vi "JSON Alarmas.vi"(0 "time":u32, 1 "high bat":dbl, 2 "Fault Modul":dbl, 5 "Temperatura":dbl, 7 "Common Sys":dbl, 9 "out line 1":dbl, 11 "error in":errorcluster, 12 "out line 3":dbl, 13 "low bat":dbl) -> (4 "alarmas":refnum<class "JSON Array.lvclass">, 15 "error out":errorcluster)   [LabVIEW 2015]
uses:
  <vilib>/addons/JSON API/Get Polymorphic/JSON GetSet.lvlib
  <vilib>/addons/JSON API/JSON Scalar/Set SGL.vi
  <vilib>/addons/JSON API/JSON Scalar/JSON Scalar.lvclass
  <vilib>/addons/JSON API/JSON Object/Set Object Item by name.vi
  <vilib>/addons/JSON API/JSON Object/JSON Object.lvclass
  <vilib>/addons/JSON API/JSON Scalar/Set String.vi
  <vilib>/addons/JSON API/JSON Array/Set JSON Array.vi
  <vilib>/addons/JSON API/JSON Array/JSON Array.lvclass
  <vilib>/addons/JSON API/JSON Scalar/Set U32.vi
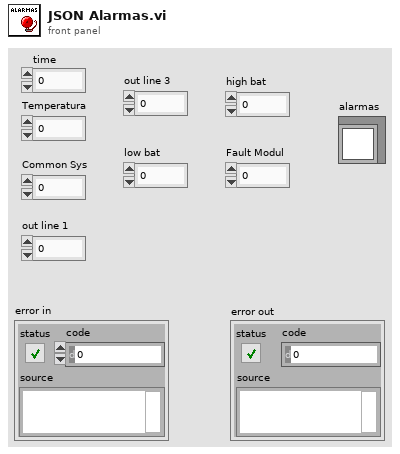
[diagram p1: front panel]
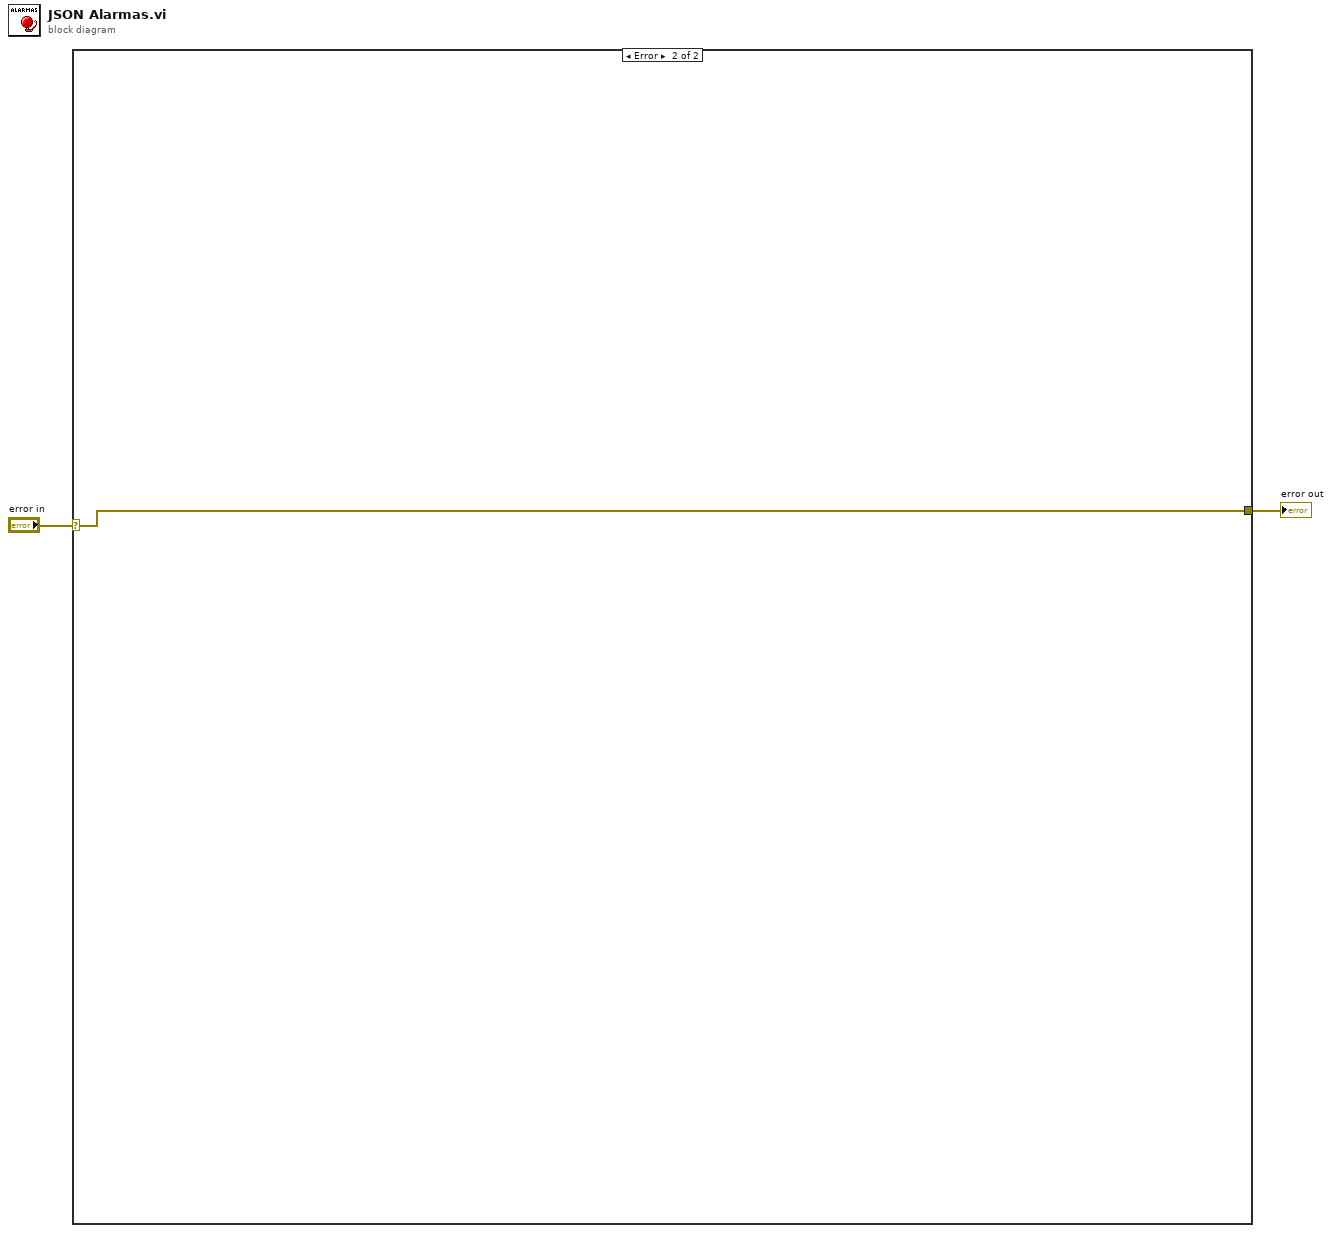
[diagram p0: block diagram]
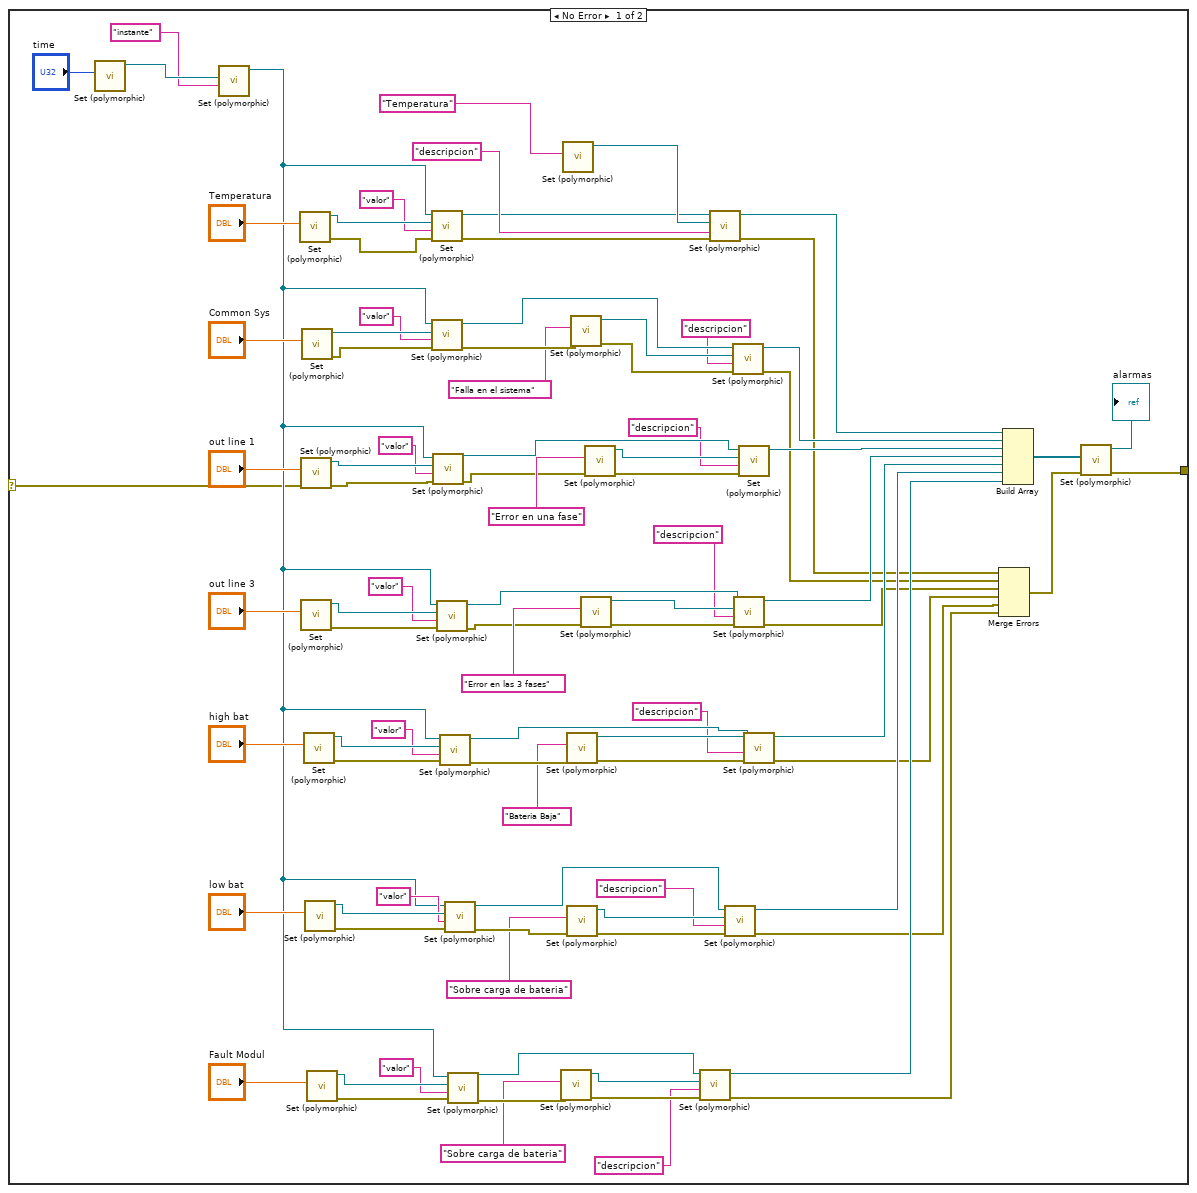
[diagram p2: hidden frame]
diagram:
  n1 = case shown="Error" "error in" {
    selector: "error in" -> [w4 w94]
    tunnel: [w5 w94] -> w2
    frame No Error {
      n2 = call-poly <vilib>:"Set (polymorphic).vi"("Numeric"="time") -> ("JSON Scalar out"=w8:refnum<class "JSON Scalar.lvclass">)  [unwired: 9 in, 1 out]
      n3 = call-poly <vilib>:"Set (polymorphic).vi"("name"="instante", "Value"=w8) -> ("JSON Object out"=w6:refnum<class "JSON Object.lvclass">)  [unwired: 7 in, 2 out]
      n4 = call-poly <vilib>:"Set (polymorphic).vi"("Numeric"="Temperatura") -> ("error out"=w79:errorcluster, "JSON Scalar out"=w86:refnum<class "JSON Scalar.lvclass">)  [unwired: 9 in]
      n5 = call-poly <vilib>:"Set (polymorphic).vi"("error in (no error)"=w4, "Numeric"="out line 1") -> ("error out"=w67:errorcluster, "JSON Scalar out"=w66:refnum<class "JSON Scalar.lvclass">)  [unwired: 8 in]
      n6 = call-poly <vilib>:"Set (polymorphic).vi"("Numeric"="out line 3") -> ("error out"=w55:errorcluster, "JSON Scalar out"=w57:refnum<class "JSON Scalar.lvclass">)  [unwired: 9 in]
      n7 = call-poly <vilib>:"Set (polymorphic).vi"("Numeric"="Common Sys") -> ("error out"=w76:errorcluster, "JSON Scalar out"=w77:refnum<class "JSON Scalar.lvclass">)  [unwired: 9 in]
      n8 = call-poly <vilib>:"Set (polymorphic).vi"("Numeric"="high bat") -> ("error out"=w45:errorcluster, "JSON Scalar out"=w47:refnum<class "JSON Scalar.lvclass">)  [unwired: 9 in]
      n9 = call-poly <vilib>:"Set (polymorphic).vi"("Numeric"="low bat") -> ("error out"=w35:errorcluster, "JSON Scalar out"=w37:refnum<class "JSON Scalar.lvclass">)  [unwired: 9 in]
      n10 = call-poly <vilib>:"Set (polymorphic).vi"("Numeric"="Fault Modul") -> ("error out"=w25:errorcluster, "JSON Scalar out"=w28:refnum<class "JSON Scalar.lvclass">)  [unwired: 9 in]
      n11 = call-poly <vilib>:"Set (polymorphic).vi"("error in (no error)"=w79, "name"="valor", "Value"=w86, "JSON Object in"=w6) -> ("error out"=w80:errorcluster, "JSON Object out"=w81:refnum<class "JSON Object.lvclass">)  [unwired: 5 in, 1 out]
      n12 = call-poly <vilib>:"Set (polymorphic).vi"("error in (no error)"=w76, "name"="valor", "Value"=w77, "JSON Object in"=w6) -> ("error out"=w74:errorcluster, "JSON Object out"=w71:refnum<class "JSON Object.lvclass">)  [unwired: 5 in, 1 out]
      n13 = call-poly <vilib>:"Set (polymorphic).vi"("error in (no error)"=w67, "name"="valor", "Value"=w66, "JSON Object in"=w6) -> ("error out"=w63:errorcluster, "JSON Object out"=w61:refnum<class "JSON Object.lvclass">)  [unwired: 5 in, 1 out]
      n14 = call-poly <vilib>:"Set (polymorphic).vi"("error in (no error)"=w55, "name"="valor", "Value"=w57, "JSON Object in"=w6) -> ("error out"=w50:errorcluster, "JSON Object out"=w52:refnum<class "JSON Object.lvclass">)  [unwired: 5 in, 1 out]
      n15 = call-poly <vilib>:"Set (polymorphic).vi"("error in (no error)"=w45, "name"="valor", "Value"=w47, "JSON Object in"=w6) -> ("error out"=w44:errorcluster, "JSON Object out"=w42:refnum<class "JSON Object.lvclass">)  [unwired: 5 in, 1 out]
      n16 = call-poly <vilib>:"Set (polymorphic).vi"("error in (no error)"=w35, "name"="valor", "Value"=w37, "JSON Object in"=w6) -> ("error out"=w34:errorcluster, "JSON Object out"=w27:refnum<class "JSON Object.lvclass">)  [unwired: 5 in, 1 out]
      n17 = call-poly <vilib>:"Set (polymorphic).vi"("error in (no error)"=w25, "name"="valor", "Value"=w28, "JSON Object in"=w6) -> ("error out"=w24:errorcluster, "JSON Object out"=w20:refnum<class "JSON Object.lvclass">)  [unwired: 5 in, 1 out]
      n18 = call-poly <vilib>:"Set (polymorphic).vi"("error in (no error)"=w24, "String"="Sobre carga de bateria" ("name")) -> ("error out"=w21:errorcluster, "JSON Scalar out"=w22:refnum<class "JSON Scalar.lvclass">)  [unwired: 8 in]
      n19 = call-poly <vilib>:"Set (polymorphic).vi"("String"="Temperatura" ("JSON stream")) -> ("JSON Scalar out"=w83:refnum<class "JSON Scalar.lvclass">)  [unwired: 9 in, 1 out]
      n20 = call-poly <vilib>:"Set (polymorphic).vi"("error in (no error)"=w44, "String"="Bateria Baja" ("name")) -> ("error out"=w41:errorcluster, "JSON Scalar out"=w43:refnum<class "JSON Scalar.lvclass">)  [unwired: 8 in]
      n21 = call-poly <vilib>:"Set (polymorphic).vi"("error in (no error)"=w34, "String"="Sobre carga de bateria" ("name")) -> ("error out"=w31:errorcluster, "JSON Scalar out"=w32:refnum<class "JSON Scalar.lvclass">)  [unwired: 8 in]
      n22 = call-poly <vilib>:"Set (polymorphic).vi"("error in (no error)"=w74, "String"="Falla en el sistema" ("name")) -> ("error out"=w69:errorcluster, "JSON Scalar out"=w72:refnum<class "JSON Scalar.lvclass">)  [unwired: 8 in]
      n23 = call-poly <vilib>:"Set (polymorphic).vi"("error in (no error)"=w50, "String"="Error en las 3 fases" ("name")) -> ("error out"=w49:errorcluster, "JSON Scalar out"=w53:refnum<class "JSON Scalar.lvclass">)  [unwired: 8 in]
      n24 = call-poly <vilib>:"Set (polymorphic).vi"("error in (no error)"=w63, "String"="Error en una fase" ("name")) -> ("error out"=w59:errorcluster, "JSON Scalar out"=w62:refnum<class "JSON Scalar.lvclass">)  [unwired: 8 in]
      n25 = call-poly <vilib>:"Set (polymorphic).vi"("error in (no error)"=w21, "name"="descripcion", "Value"=w22, "JSON Object in"=w20) -> ("error out"=w13:errorcluster, "JSON Object out"=w19:refnum<class "JSON Object.lvclass">)  [unwired: 5 in, 1 out]
      n26 = call-poly <vilib>:"Set (polymorphic).vi"("error in (no error)"=w80, "name"="descripcion", "Value"=w83, "JSON Object in"=w81) -> ("error out"=w18:errorcluster, "JSON Object out"=w78:refnum<class "JSON Object.lvclass">)  [unwired: 5 in, 1 out]
      n27 = call-poly <vilib>:"Set (polymorphic).vi"("error in (no error)"=w31, "name"="descripcion", "Value"=w32, "JSON Object in"=w27) -> ("error out"=w14:errorcluster, "JSON Object out"=w29:refnum<class "JSON Object.lvclass">)  [unwired: 5 in, 1 out]
      n28 = call-poly <vilib>:"Set (polymorphic).vi"("error in (no error)"=w69, "name"="descripcion", "Value"=w72, "JSON Object in"=w71) -> ("error out"=w17:errorcluster, "JSON Object out"=w70:refnum<class "JSON Object.lvclass">)  [unwired: 5 in, 1 out]
      n29 = call-poly <vilib>:"Set (polymorphic).vi"("error in (no error)"=w49, "name"="descripcion", "Value"=w53, "JSON Object in"=w52) -> ("error out"=w16:errorcluster, "JSON Object out"=w48:refnum<class "JSON Object.lvclass">)  [unwired: 5 in, 1 out]
      n30 = call-poly <vilib>:"Set (polymorphic).vi"("error in (no error)"=w59, "name"="descripcion", "Value"=w62, "JSON Object in"=w61) -> ("JSON Object out"=w58:refnum<class "JSON Object.lvclass">)  [unwired: 5 in, 2 out]
      n31 = call-poly <vilib>:"Set (polymorphic).vi"("error in (no error)"=w41, "name"="descripcion", "Value"=w43, "JSON Object in"=w42) -> ("error out"=w15:errorcluster, "JSON Object out"=w39:refnum<class "JSON Object.lvclass">)  [unwired: 5 in, 1 out]
      n32 = Merge Errors(w18, w17, w16, w15, w14, w13) -> (w10:errorcluster)
      n33 = Build Array(w78, w70, w58, w48, w39, w29, w19) -> (w11:refnum<class "JSON Object.lvclass">[])
      n34 = call-poly <vilib>:"Set (polymorphic).vi"("error in (no error)"=w10, "Array"=w11) -> ("error out"=w5:errorcluster, "JSON Array out"=→"alarmas":refnum<class "JSON Array.lvclass">)  [unwired: 8 in]
    }
    frame Error {
    }
  }
  "error out" <- w2
